vi "Layout.vi"(0 "Slide in":refnum<vi>, 5 "D space":refnum<vi>, 9 "NewBnds":T1) -> ()   [LabVIEW 2020, in "DiskSpaceMonitor.xctl"]
uses:
  DiskSpaceMonitor.xctl
  <vilib>/Utility/miscctls.llb/LVRectTypeDef.ctl
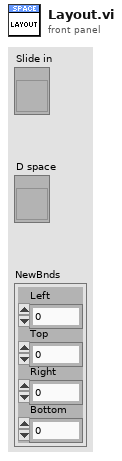
[diagram p1: front panel]
types:
  T1 = typedef "LVRectTypeDef.ctl" = cluster{"Left":i16, "Top":i16, "Right":i16, "Bottom":i16}
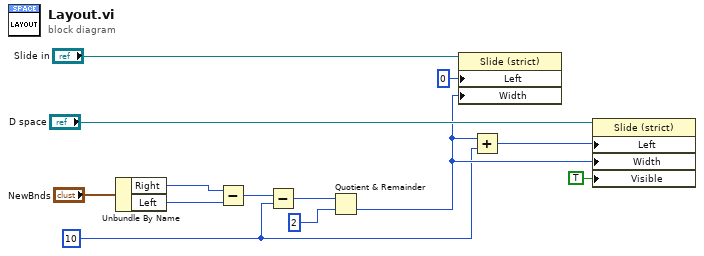
[diagram p0: block diagram]
diagram:
  w3 = i16 10 ("y")
  n1 = Unbundle By Name("NewBnds") -> ("Right"=w12:i16, "Left"=w11:i16)
  n2 = Subtract(x=w12, y=w11) -> (x-y=w10:i16)
  n3 = Subtract(x=w10, y=w3) -> (x-y=w9:i16)
  n4 = Quotient & Remainder(x=w9, y=i16 2) -> (floor(x/y)=w4:i16)  [unwired: 1 out]
  n5 = property class="Slide (strict)"(reference="Slide in", "Left"=0 ("Position:Left"), "Width"=w4) -> ()  [unwired: 1 in, 2 out]
  n6 = Add(x=w4, y=w3) -> (x+y=w2:i16)
  n7 = property class="Slide (strict)"(reference="D space", "Left"=w2, "Width"=w4, "Visible"=TRUE) -> ()  [unwired: 1 in, 2 out]
